vi "GOMBDTS2048 big sample.vi"() -> ()   [LabVIEW 2009]
uses:
  <vilib>/Utility/miscctls.llb/LVComboBoxStrsAndValuesArrayTypeDef.ctl
  <vilib>/Utility/file.llb/Write To Spreadsheet File (string).vi
panel:
  out "date/time string":string
  in  "Tab Control":T1(tab)
  in  "Configuration":string(combo)
  in  "Save Measurement":bool
  in  "Start Measurement":bool
  in  "Stop Software":bool
  in  "Initialize":bool
  out "XY Graph":cluster{"lambdas":dbl[], "counts":dbl[]}(graph)
  in  "X-Achse":enum16{"Wellenlänge / nm", "Pixel"}(ring)
  out "Filterposition":i32
  out "spectral unit":string
  out "integral unit":string
  out "x":dbl
  out "y":dbl
  out "T":dbl
  out "us":dbl
  out "vs":dbl
  out "domWL":dbl
  out "lambda peak":dbl
  out "fwhm":dbl
  out "scaling factor diode":dbl
  out "T / °C":dbl
  out "UpperX":dbl
  out "UpperY":dbl
  out "UpperZ":dbl
  out "Werte Y-Achse":dbl[](array[numeric])
  out "Werte X-Achse":dbl[](array[numeric])
  in  "Integrationszeit Automatisch?":bool=TRUE
  out "Integrationszeit / us":i32
  in  "Bandbreitenkorrektur":bool
  in  "Linearitätskorrektur":bool
  in  "a(Z)":bool
  in  "scale by diode":bool
  in  "Savitzky \nGolay Filter":bool
  out "az":dbl
  in  "Messmodus":T2(ring)
  in  "Anzahl Mittelungen":i32=1
  in  "Integrationszeit manuell / us":i32
  out "Temperature / °C":dbl
  in  "serial number device":string
  out "Integral value":dbl format="%#_6e"
  out "uv":dbl
  out "power peak":dbl
  out "handle":i32
  in  "Dateiname Selbstabsorptionskorrektur":string="sub1.gsc"
  in  "Selbstabsorptions-Korrektur nutzen?":bool
  in  "Speicherpfad Selbstabsorptions-Korrektur":path
  out "substititution factors array":dbl[](array[numeric])
  out "substitution factor diode":dbl
  out "function return 1":i32
  out "function return 3":i32
  out "Array function return 4":i32[](array[numeric])
  out "function return 5":i32
  out "function return 6":i32
  out "function return 7":i32
  out "function return 8":i32
  out "function return 14":i32
  out "function return 15":i32
  out "function return 16":i32
  out "function return 17":i32
  out "function return 19":i32
  out "function return 20":i32
  out "function return 21":i32
  out "function return 22":i32
  out "function return 23":i32
  out "function return 24":i32
  out "function return 25":i32
  out "function return 26":i32
  out "function return 27":i32
  out "function return 28":i32
  out "function return 29":i32
  out "function return 31":i32
  out "function return 34":i32
  out "function return 35":i32
  out "function return 36":i32
  out "function return 37":i32
  out "function return 38":i32
  out "function return 39":i32
  out "function return 40":i32
  out "function return 41":i32
  out "function return 43":i32
  out "function return 44":i32
  out "function return 45":i32
  out "function return 30":i32
  out "function return 33":i32
  out "function return 11":i32
  out "function return 10":i32
  out "function return 42":i32
  out "function return 32":i32
  out "function return 12":i32
  out "function return 13":i32
  out "function return 18":i32
  in  "error in":errorcluster
  out "error out":errorcluster
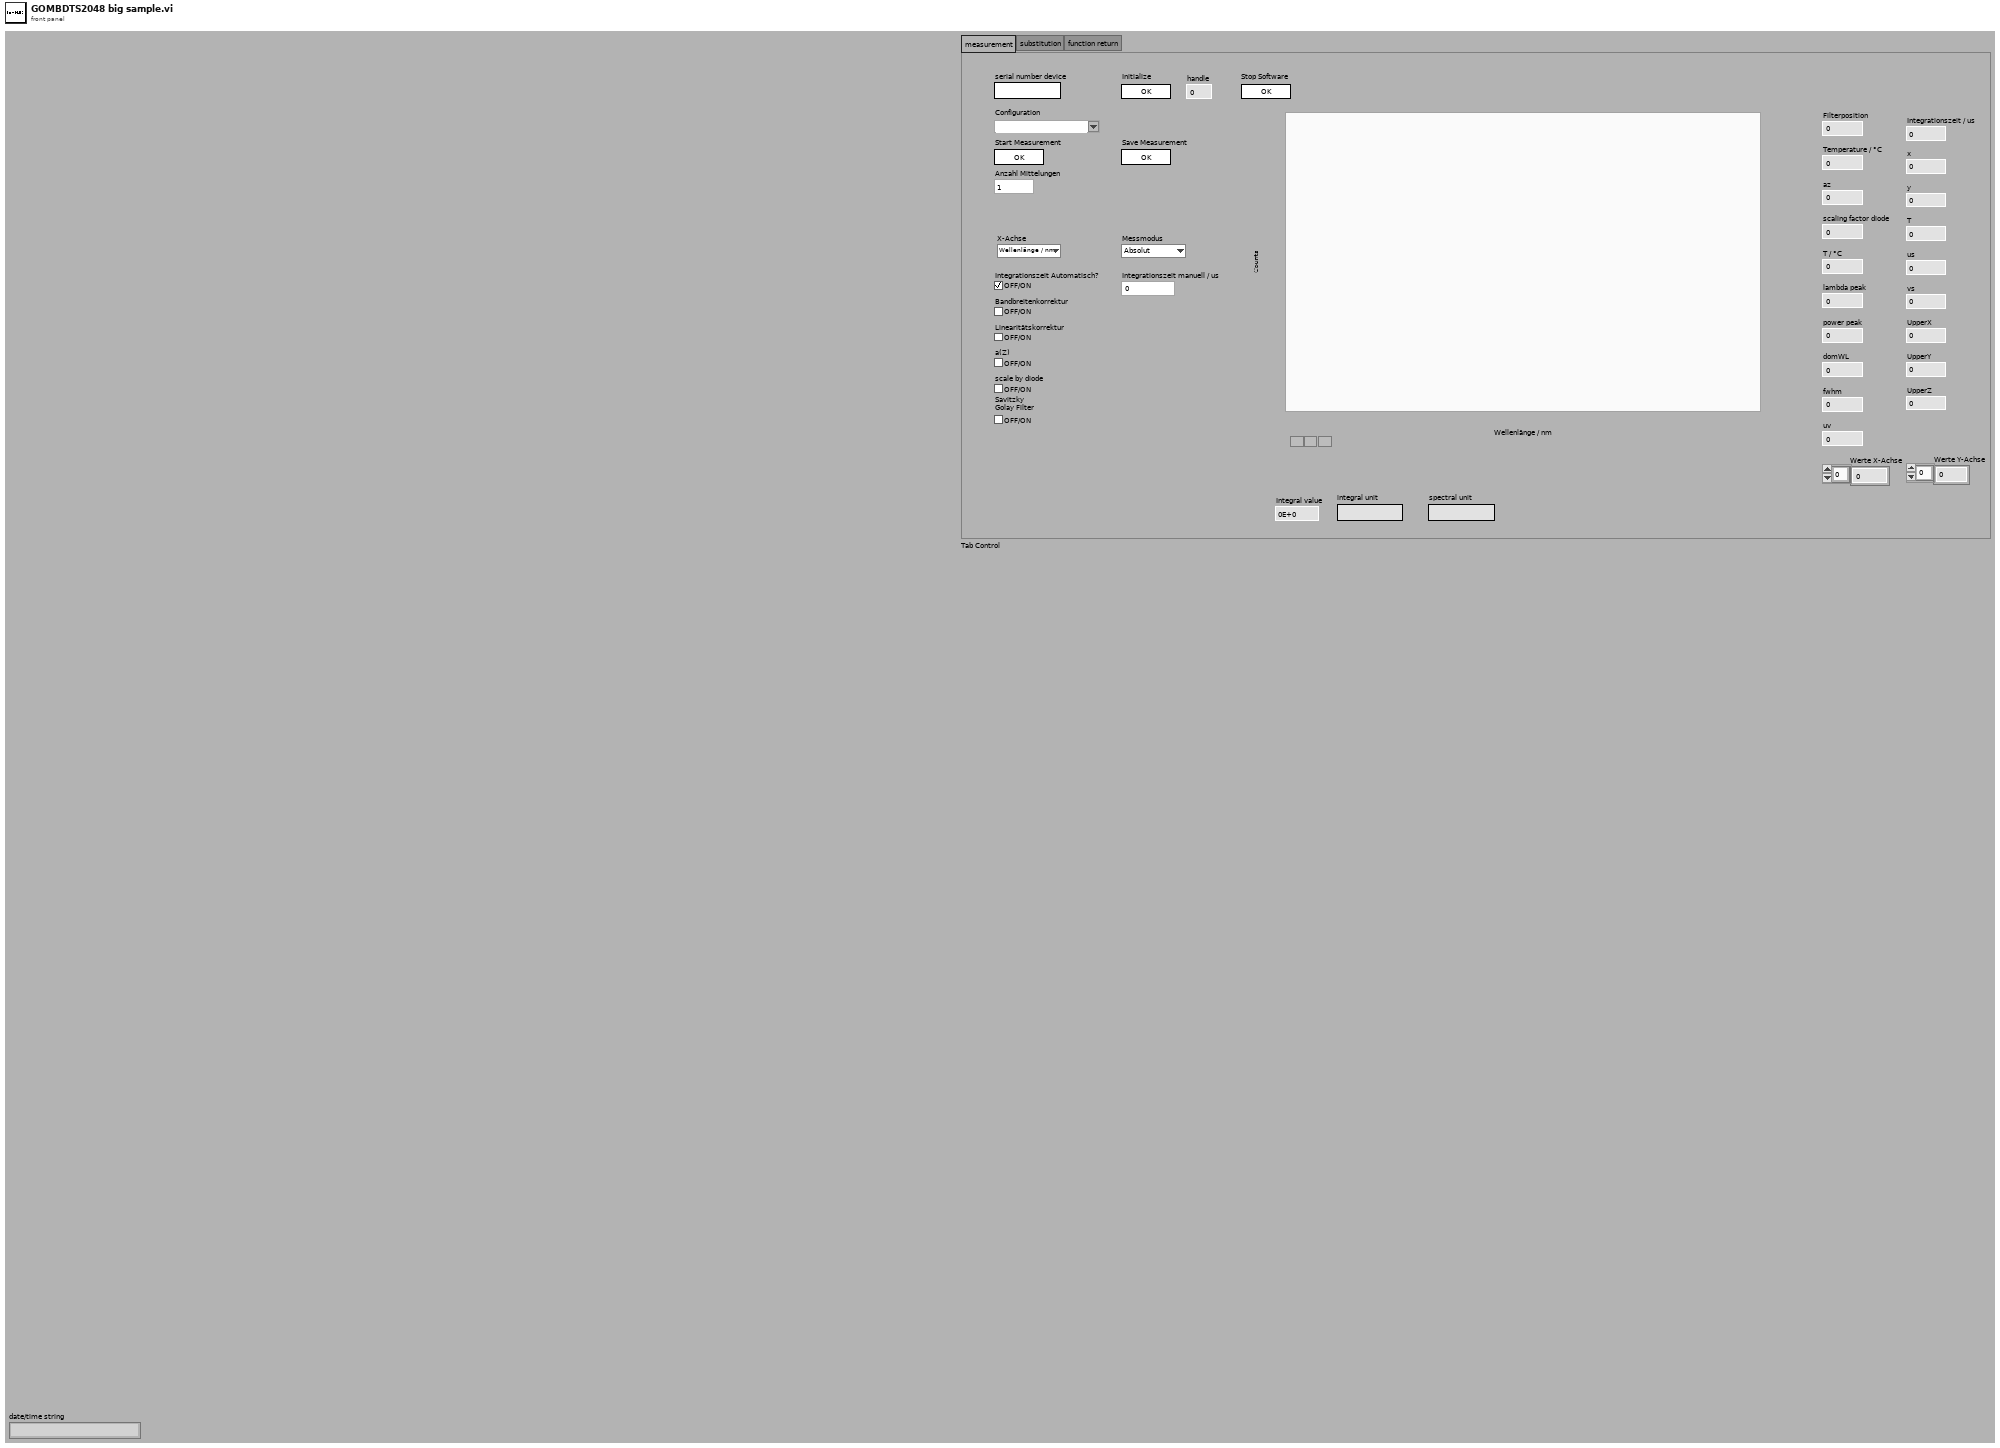
[diagram p1: front panel]
types:
  T1 = enum32{"measurement", "substitution", "function return"}
  T2 = enum16{"Absolut", "Counts", "Counts nur Hell", "Counts nur Dunkel"}
  T3 = typedef "LVComboBoxStrsAndValuesArrayTypeDef.ctl" = cluster{"String":string, "Value":string}[]
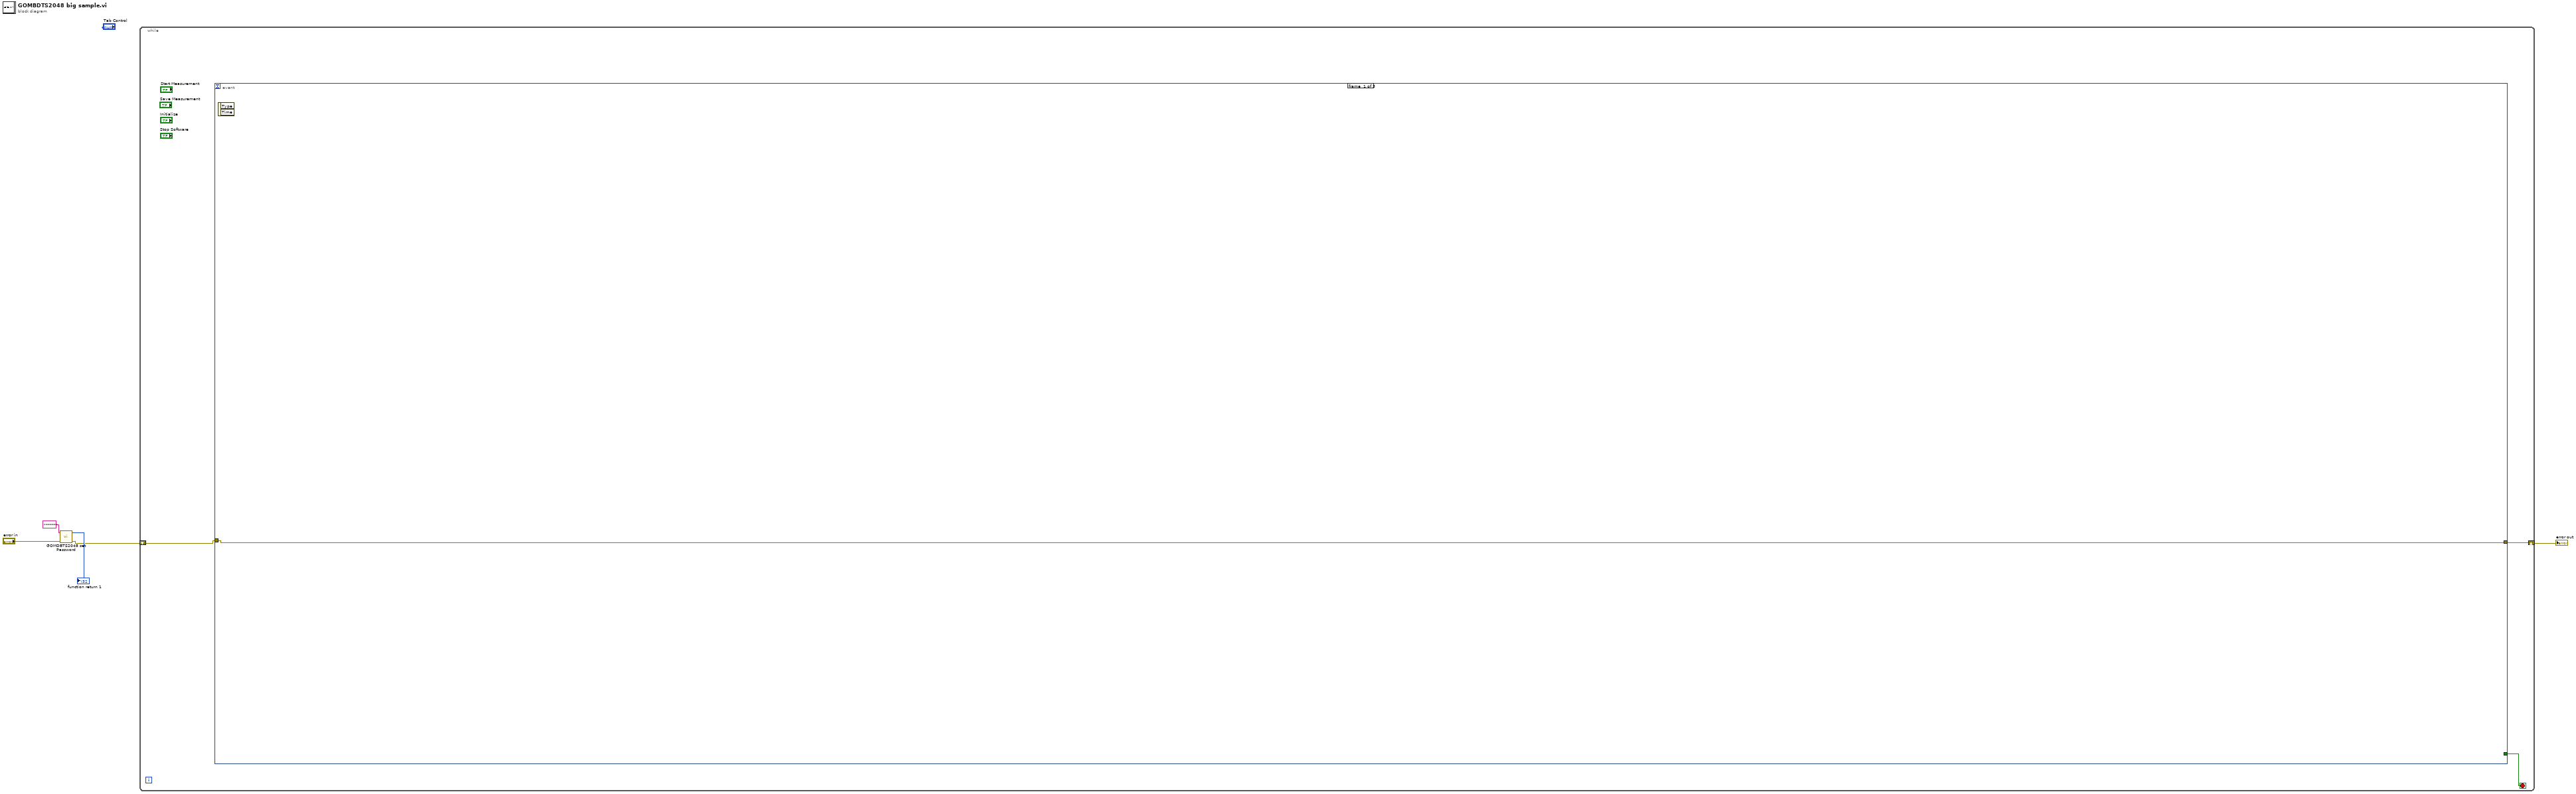
[diagram p0: block diagram]
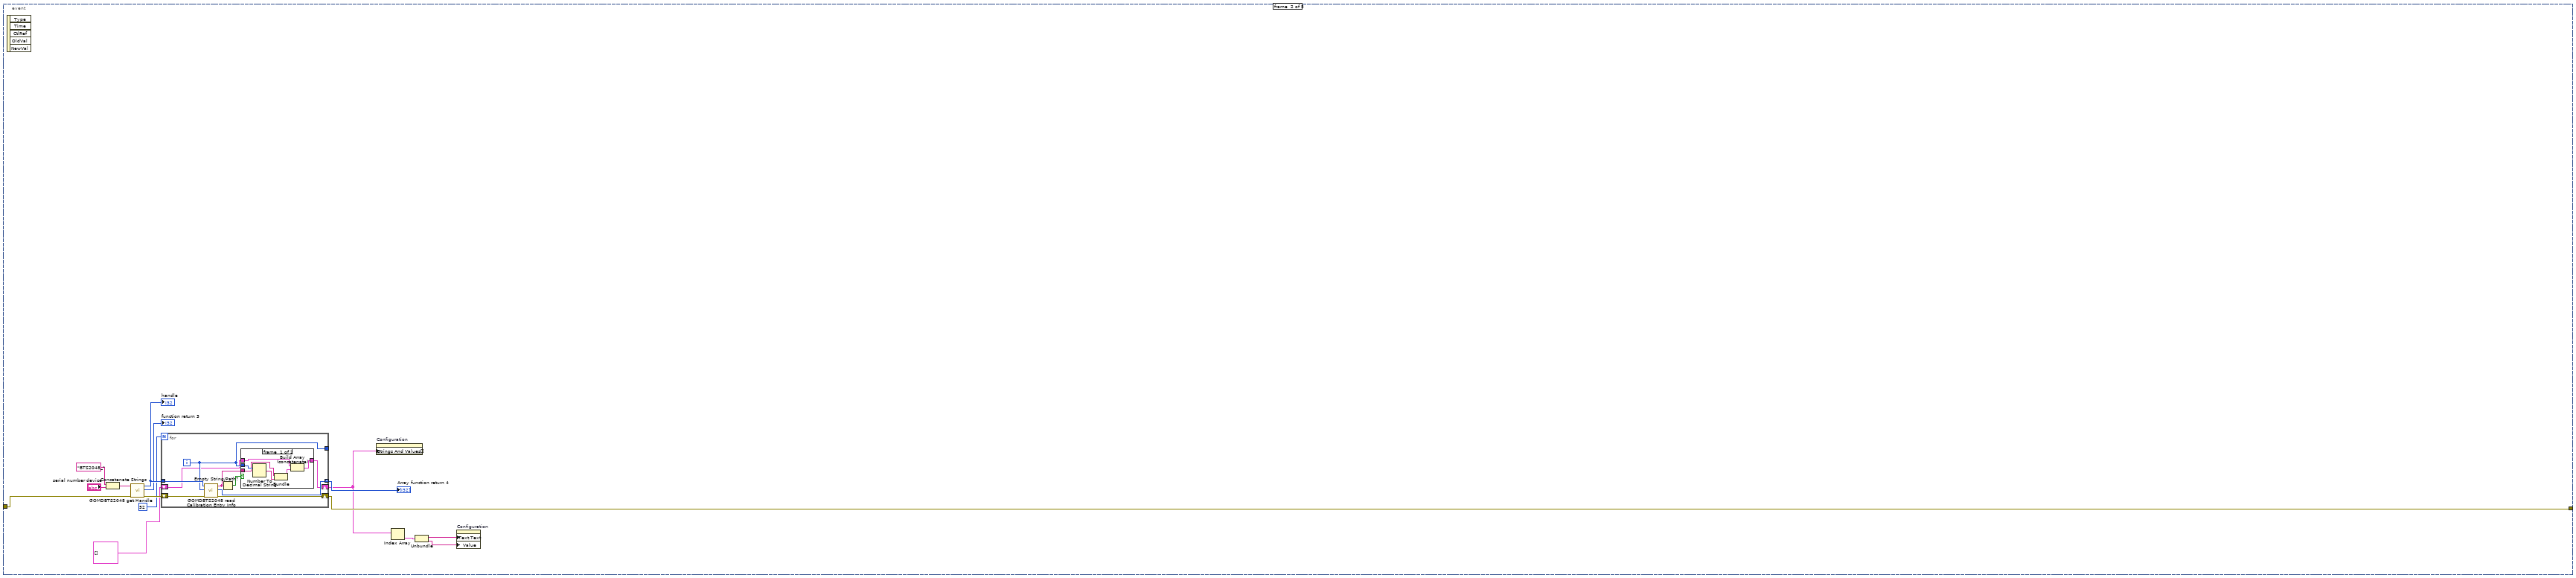
[diagram p2: hidden frame]
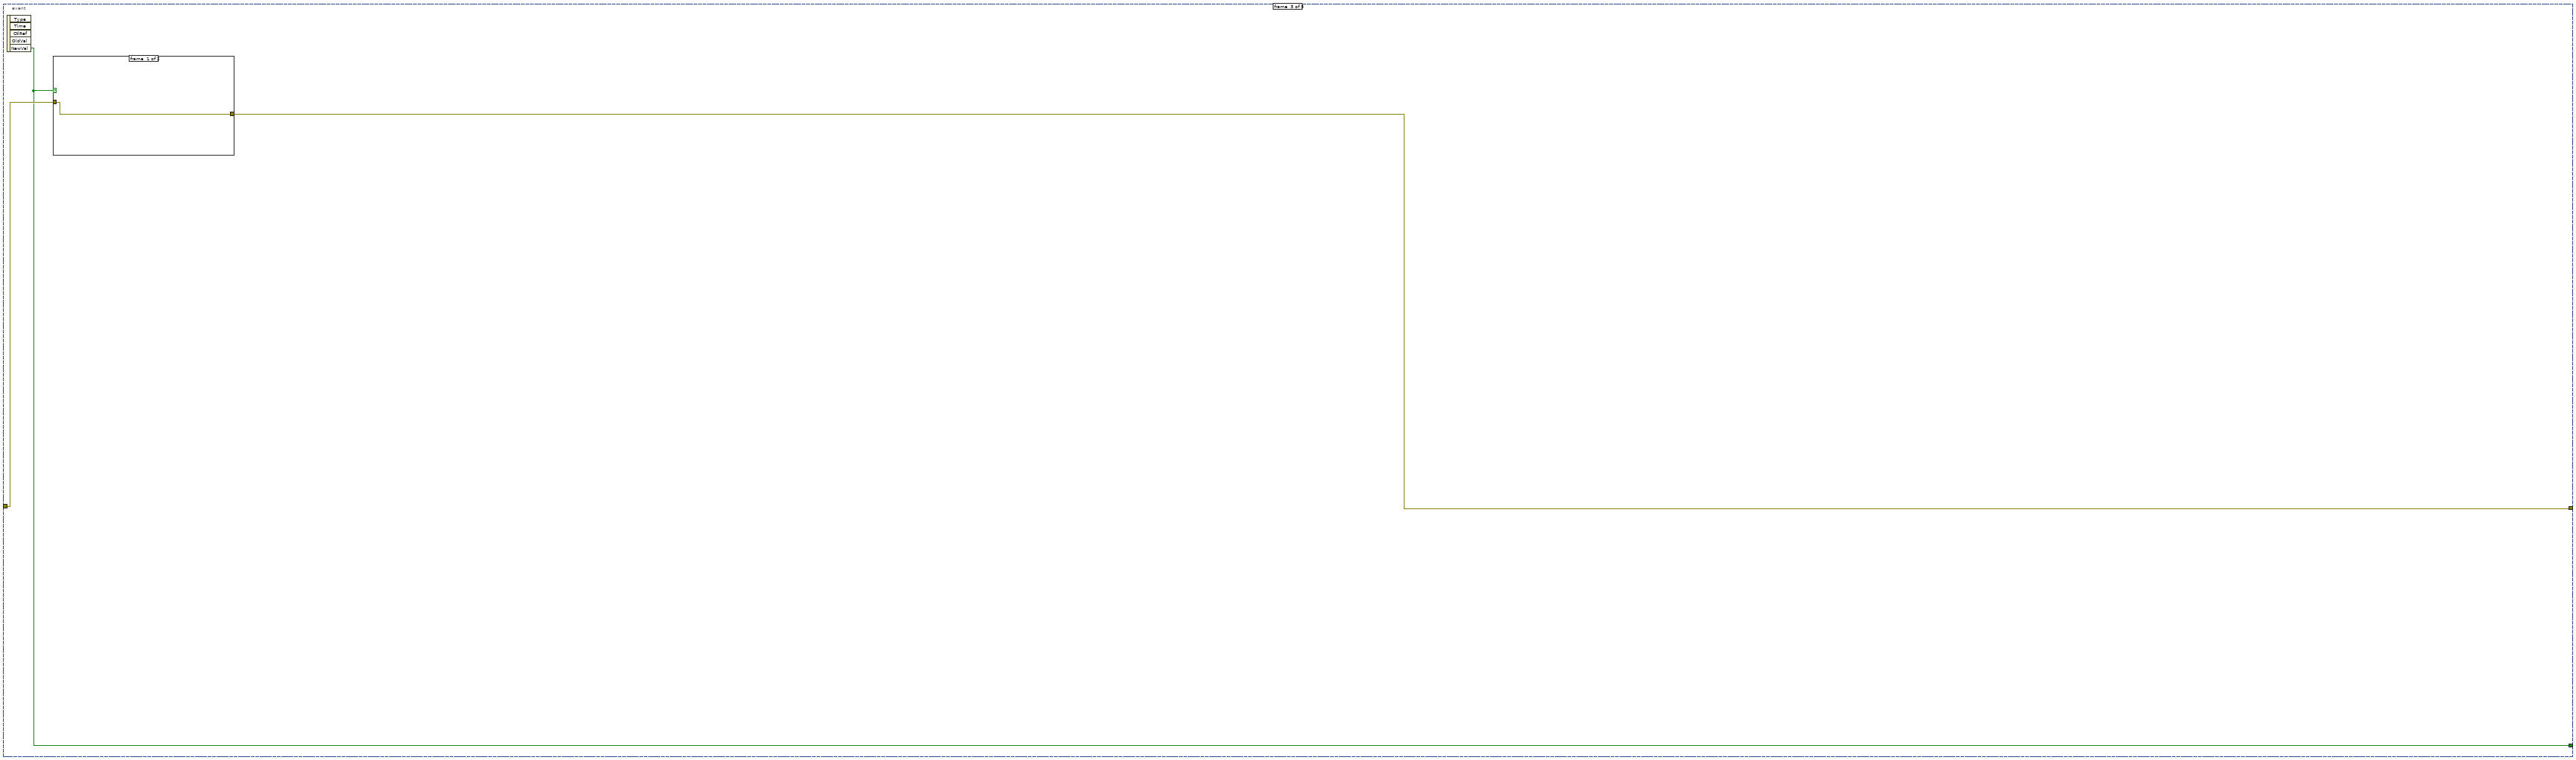
[diagram p4: hidden frame]
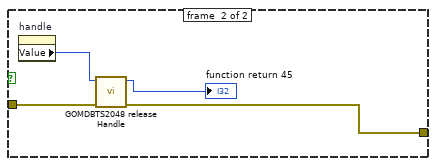
[diagram p5: hidden frame]
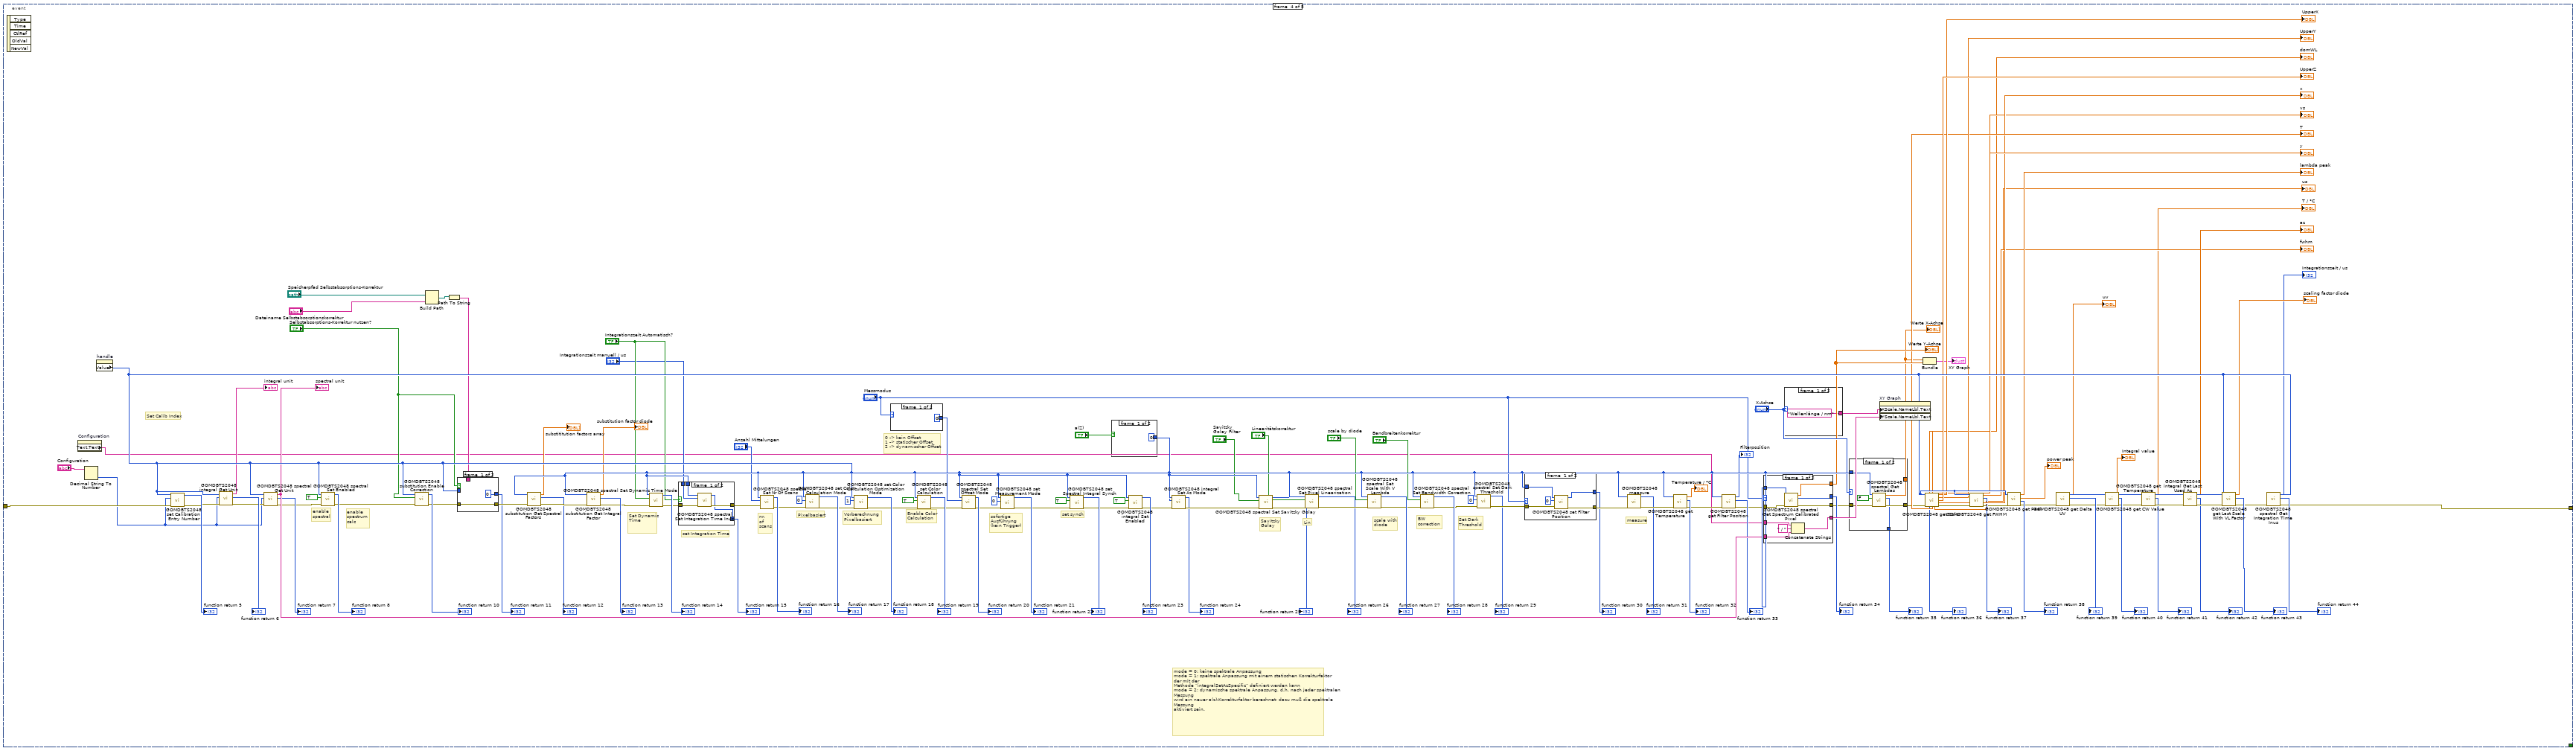
[diagram p6: hidden frame]
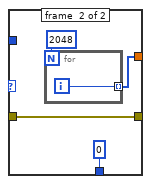
[diagram p7: hidden frame]
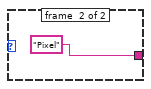
[diagram p8: hidden frame]
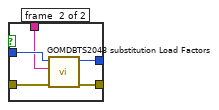
[diagram p9: hidden frame]
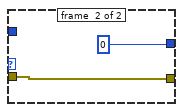
[diagram p10: hidden frame]
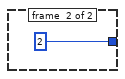
[diagram p11: hidden frame]
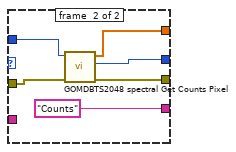
[diagram p12: hidden frame]
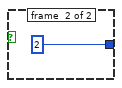
[diagram p13: hidden frame]
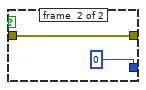
[diagram p14: hidden frame]
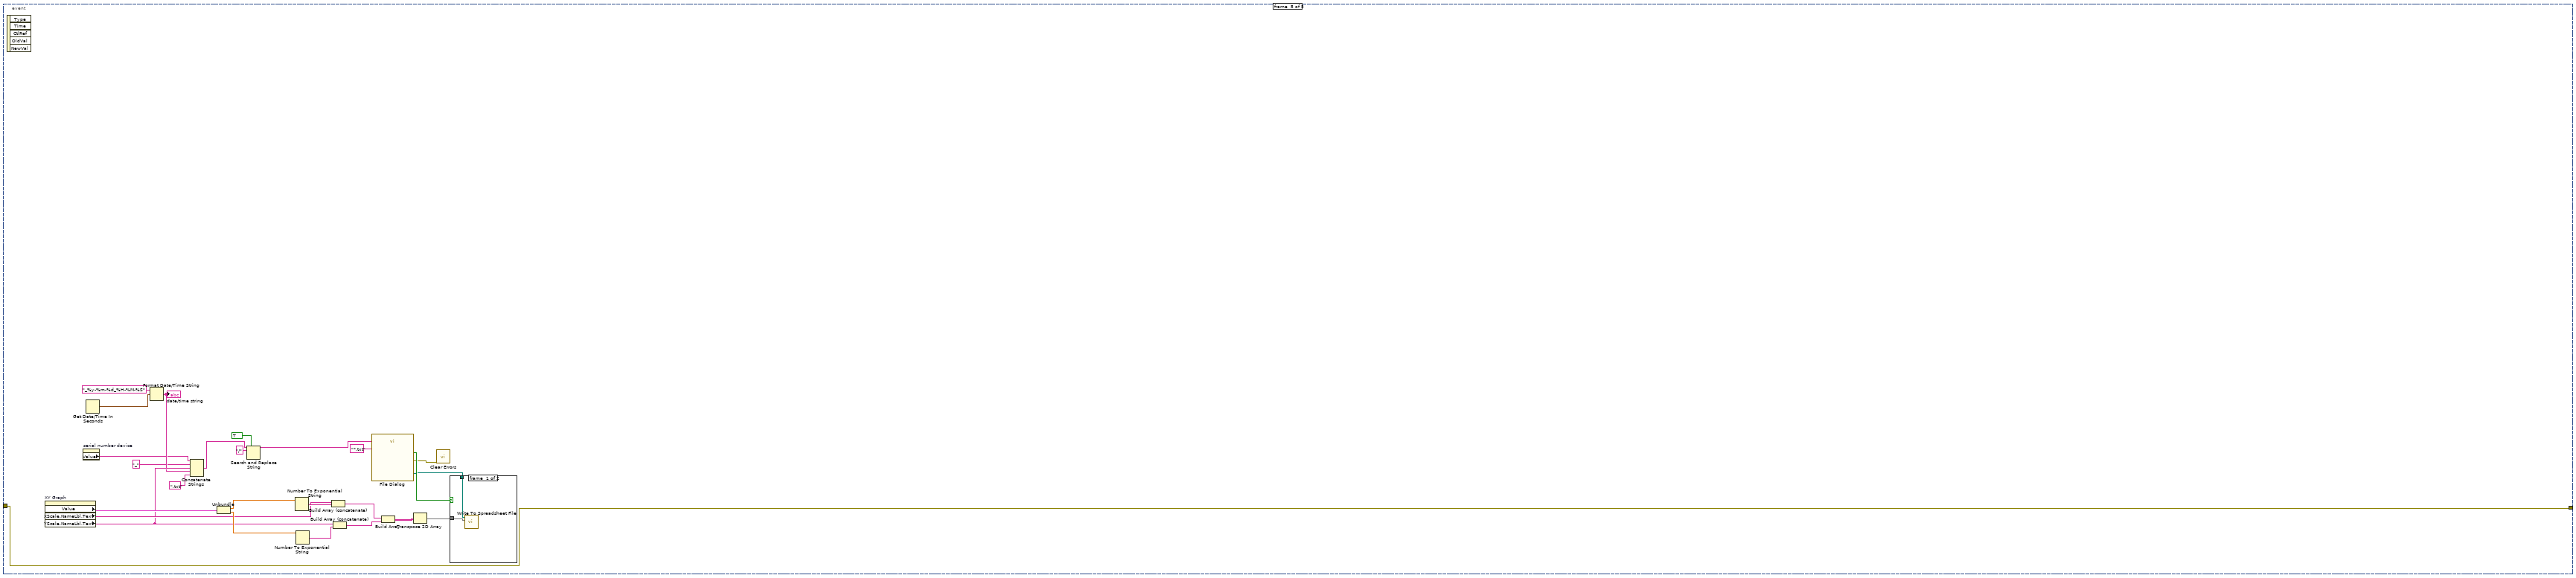
[diagram p15: hidden frame]
diagram:
  n1 = call <userlib>:"GOMDBTS2048 set Password.vi"("error in (no error)"="error in", "value"="*****" ("Password")) -> ("error out"=w2:errorcluster, "function return"=→"function return 1":i32)  [unwired: 8 in]
  n2 = while {
    shift-right: [w7] -> w1
    shift-left: w2 -> [w8]
    stop <- w6 stop-if-true
    n3 = event shown="[3] \"Start Measurement\": Value Change" {
      selector: _ -> [_ _ _ _ _]
      dyn-events: _ -> [_ _ _ _ _]
      timeout: _ -> [_ _ _ _ _]
      tunnel: w8 -> [w9 w16 w43 w57 w246]
      tunnel: [w9 w15 w42 w56 w246] -> w7
      tunnel: [_ _ w41 _ _] -> w6
      event #0 {
        n4 = event-data() -> ()  [unwired: 1 in, 2 out]
      }
      event #1 {
        n5 = event-data() -> ()  [unwired: 1 in, 5 out]
        n6 = Concatenate Strings("BTS2048_", "serial number device") -> (w18:string)
        n7 = call <userlib>:"GOMDBTS2048 get Handle.vi"("error in (no error)"=w16, "device"=w18) -> ("error out"=w20:errorcluster, "function return"=→"function return 3":i32, "handle"=w24:i32)  [unwired: 7 in]
        "handle" <- w24
        n8 = for {
          N: 52 -> [_]
          shift-right: [w31] -> w15
          shift-left: w20 -> [w32]
          tunnel: w24 -> [w33]
          tunnel: [w29] -> _
          tunnel: [w30] -> w22 mode=indexing
          shift-right: [w26] -> w13
          shift-left: T3 [] ("Strings And Values []") -> [w25]
          i -> [w29]
          n9 = call <userlib>:"GOMDBTS2048 read Calibration Entry Info.vi"("error in (no error)"=w32, "calibrationEntryNumber"=w29, "handle"=w33) -> ("error out"=w31:errorcluster, "function return"=w30:i32, "calibrationName"=w28:string)  [unwired: 6 in]
          n10 = Empty String/Path?(string/path=w28) -> (empty?=w27:bool)
          n11 = case shown="False" w27 {
            tunnel: w29 -> [w39 _]
            tunnel: w28 -> [w36 _]
            tunnel: [w37 w40] -> w26
            tunnel: w25 -> [w38 w40]
            frame #0 {
              n12 = Number To Decimal String(number=w39) -> (decimal integer string=w35:string)  [unwired: 1 in]
              n13 = Bundle("calibrationName"=w36, w35) -> (w34:cluster{"calibrationName":string, string})  [unwired: 1 in]
              n14 = Build Array (concatenate)(w38, w34) -> (w37:T3)
            }
            frame #1 {
            }
          }
        }
        "Array function return 4" <- w22
        n15 = property on="Configuration" class="CmbBox"("Strings And Values[]"=w13) -> ()  [unwired: 2 in, 2 out]
        n16 = Index Array(array=w13) -> (element=w12:cluster{"String":string, "Value":string})  [unwired: 1 in]
        n17 = Unbundle(w12) -> ("String"=w11:string, "Value"=w10:string)
        n18 = property on="Configuration" class="CmbBox"("Text.Text"=w11, "Value"=w10) -> ()  [unwired: 2 in, 2 out]
      }
      event #2 {
        n19 = event-data() -> ("NewVal"=w41:bool)  [unwired: 1 in, 4 out]
        n20 = case shown="True" w41 {
          tunnel: w43 -> [w44 w48]
          tunnel: [w44 w47] -> w42
          frame #0 {
          }
          frame #1 {
            n21 = property on="handle" class="DigNum (strict)"() -> ("Value"=w45:i32)  [unwired: 2 in, 2 out]
            n22 = call <userlib>:"GOMDBTS2048 release Handle.vi"("error in (no error)"=w48, "handle"=w45) -> ("error out"=w47:errorcluster, "function return"=→"function return 45":i32)  [unwired: 8 in]
          }
        }
      }
      event #3 {
        # "measure"
        # "Set Dark\nThreshold"
        # "BW \ncorrection"
        # "scale with\ndiode"
        # "Lin"
        # "Savitzky \nGolay"
        # "nr. \nof \nscans"
        # "enable\nspectrum\ncalc"
        # "enable\nspectral"
        # "set synch"
        # "sofortige\nAusführung\n(kein Trigger)"
        # "mode = 0: keine spektrale Anpassung\nmode = 1: spektrale Anpassung mit einem statischen Korrekturfaktor der mit der\nMethode “integralSetAzSpecific” definiert werden kann\nmode = 2: dynamische spektrale Anpassung, d.h. nach jeder spektralen Messung\nwird ein neuer a(z)-Korrekturfaktor berechnet; dazu muß die spektrale Messung\naktiviert sein."
        # "0 -> kein Offset\n1 -> statischer Offset\n2 -> dynamischer Offset"
        # "Set Calib Index"
        # "Set Dynamic Time"
        # "set Integration Time"
        # "Enable Color\nCalculation"
        # "Vorberechnung \nPixelbasiert"
        # "Pixelbasiert"
        n23 = event-data() -> ()  [unwired: 1 in, 5 out]
        n24 = property on="Configuration" class="CmbBox"() -> ("Text.Text"=w53:string)  [unwired: 2 in, 2 out]
        n25 = Decimal String To Number(string="Configuration") -> (number=w54:i32)  [unwired: 2 in, 1 out]
        n26 = property on="handle" class="DigNum (strict)"() -> ("Value"=w185:i32)  [unwired: 2 in, 2 out]
        n27 = call <userlib>:"GOMDBTS2048 set Calibration Entry Number.vi"("error in (no error)"=w57, "calibrationEntryNumber"=w54, "handle"=w185) -> ("error out"=w86:errorcluster, "function return"=→"function return 5":i32)  [unwired: 7 in]
        n28 = call <userlib>:"GOMDBTS2048 integral Get Unit.vi"("error in (no error)"=w86, "calibrationEntryNumber"=w54, "handle"=w185) -> ("error out"=w87:errorcluster, "function return"=→"function return 6":i32, "unit"=→"integral unit":string)  [unwired: 6 in]
        n29 = call <userlib>:"GOMDBTS2048 spectral Get Unit.vi"("error in (no error)"=w87, "calibrationEntryNumber"=w54, "handle"=w185) -> ("error out"=w88:errorcluster, "function return"=→"function return 7":i32, "unit"=w183:string)  [unwired: 6 in]
        "spectral unit" <- w183
        n30 = call <userlib>:"GOMDBTS2048 spectral Set Enabled.vi"("error in (no error)"=w88, "enabled"=TRUE, "handle"=w185) -> ("error out"=w49:errorcluster, "function return"=→"function return 8":i32)  [unwired: 7 in]
        n31 = call <userlib>:"GOMDBTS2048 substitution Enable Correction.vi"("error in (no error)"=w49, "active"="Selbstabsorptions-Korrektur nutzen?", "handle"=w185) -> ("error out"=w140:errorcluster, "function return"=→"function return 10":i32)  [unwired: 7 in]
        n32 = Build Path(base path="Speicherpfad Selbstabsorptions-Korrektur", name or relative path="Dateiname Selbstabsorptionskorrektur") -> (appended path=w143:path)
        n33 = Path To String(path=w143) -> (string=w144:string)
        n34 = case shown="True" "Selbstabsorptions-Korrektur nutzen?" {
          tunnel: w140 -> [w200 w205]
          tunnel: w185 -> [_ w204]
          tunnel: [w200 w203] -> w156
          tunnel: w144 -> [_ w202]
          tunnel: [0 ("function return") w201] -> w146
          frame #0 {
          }
          frame #1 {
            n35 = call <userlib>:"GOMDBTS2048 substitution Load Factors.vi"("error in (no error)"=w205, "absoluteFileName"=w202, "handle"=w204) -> ("error out"=w203:errorcluster, "function return"=w201:i32)  [unwired: 7 in]
          }
        }
        "function return 11" <- w146
        n36 = call <userlib>:"GOMDBTS2048 substitution Get Spectral Factors.vi"("error in (no error)"=w156, "handle"=w185) -> ("error out"=w159:errorcluster, "function return"=→"function return 12":i32, "factor"=→"substititution factors array":dbl[])  [unwired: 7 in]
        n37 = call <userlib>:"GOMDBTS2048 substitution Get Integral Factor.vi"("error in (no error)"=w159, "handle"=w185) -> ("error out"=w160:errorcluster, "function return"=→"function return 13":i32, "factor"=→"substitution factor diode":dbl)  [unwired: 7 in]
        n38 = call <userlib>:"GOMDBTS2048 spectral Set Dynamic Time Mode.vi"("error in (no error)"=w160, "value"="Integrationszeit Automatisch?", "handle"=w185) -> ("error out"=w64:errorcluster, "function return"=→"function return 14":i32)  [unwired: 7 in]
        n39 = case shown="True" "Integrationszeit Automatisch?" {
          tunnel: w64 -> [w236 w238]
          tunnel: [w235 w238] -> w80
          tunnel: w185 -> [w234 _]
          tunnel: "Integrationszeit manuell / us" -> [w233 _]
          tunnel: [w232 0 ("function return")] -> w107
          frame #0 {
            n40 = call <userlib>:"GOMDBTS2048 spectral Set Integration Time Inus.vi"("error in (no error)"=w236, "timeInus"=w233, "handle"=w234) -> ("error out"=w235:errorcluster, "function return"=w232:i32)  [unwired: 7 in]
          }
          frame #1 {
          }
        }
        "function return 15" <- w107
        n41 = call <userlib>:"GOMDBTS2048 spectral Set Nr Of Scans.vi"("error in (no error)"=w80, "value"="Anzahl Mittelungen", "handle"=w185) -> ("error out"=w81:errorcluster, "function return"=→"function return 16":i32)  [unwired: 7 in]
        n42 = call <userlib>:"GOMDBTS2048 set Color Calculation Mode.vi"("error in (no error)"=w81, "value"=0, "handle"=w185) -> ("error out"=w65:errorcluster, "function return"=→"function return 17":i32)  [unwired: 7 in]
        n43 = call <userlib>:"GOMDBTS2048 set Color Calculation Optimization Mode.vi"("error in (no error)"=w65, "value"=1, "handle"=w185) -> ("error out"=w66:errorcluster, "function return"=→"function return 18":i32)  [unwired: 7 in]
        n44 = case shown="\"Absolut\", \"Counts\"" "Messmodus" {
          tunnel: [0 ("mode") 2 ("mode")] -> w101
          frame #0 {
          }
          frame #1 {
          }
        }
        n45 = call <userlib>:"GOMDBTS2048 set Color Calculation.vi"("error in (no error)"=w66, "value"=TRUE, "handle"=w185) -> ("error out"=w70:errorcluster, "function return"=→"function return 19":i32)  [unwired: 7 in]
        n46 = call <userlib>:"GOMDBTS2048 spectral Set Offset Mode.vi"("error in (no error)"=w70, "value"=w101, "handle"=w185) -> ("error out"=w75:errorcluster, "function return"=→"function return 20":i32)  [unwired: 7 in]
        n47 = call <userlib>:"GOMDBTS2048 set Measurement Mode.vi"("error in (no error)"=w75, "measurementMode"=0, "handle"=w185) -> ("error out"=w77:errorcluster, "function return"=→"function return 21":i32)  [unwired: 7 in]
        n48 = call <userlib>:"GOMDBTS2048 set Spectral Integral Synch.vi"("error in (no error)"=w77, "value"=TRUE, "handle"=w185) -> ("error out"=w78:errorcluster, "function return"=→"function return 22":i32)  [unwired: 7 in]
        n49 = case shown="True" "a(Z)" {
          tunnel: [0 ("mode") 2 ("mode")] -> w74
          frame #0 {
          }
          frame #1 {
          }
        }
        n50 = call <userlib>:"GOMDBTS2048 integral Set Enabled.vi"("error in (no error)"=w78, "enabled"=TRUE, "handle"=w185) -> ("error out"=w73:errorcluster, "function return"=→"function return 23":i32)  [unwired: 7 in]
        n51 = call <userlib>:"GOMDBTS2048 integral Set Az Mode.vi"("error in (no error)"=w73, "mode"=w74, "handle"=w185) -> ("error out"=w175:errorcluster, "function return"=→"function return 24":i32)  [unwired: 7 in]
        n52 = call <userlib>:"GOMDBTS2048 spectral Set Savitzky Golay.vi"("error in (no error)"=w175, "value"="Savitzky \nGolay Filter", "handle"=w185) -> ("error out"=w82:errorcluster, "function return"=→"function return 25":i32)  [unwired: 7 in]
        n53 = call <userlib>:"GOMDBTS2048 spectral Set Pixel Linearization.vi"("error in (no error)"=w82, "value"="Linearitätskorrektur", "handle"=w185) -> ("error out"=w163:errorcluster, "function return"=→"function return 26":i32)  [unwired: 7 in]
        n54 = call <userlib>:"GOMDBTS2048 spectral Set Scale With V Lambda.vi"("error in (no error)"=w163, "value"="scale by diode", "handle"=w185) -> ("error out"=w83:errorcluster, "function return"=→"function return 27":i32)  [unwired: 7 in]
        n55 = call <userlib>:"GOMDBTS2048 spectral Set Bandwidth Correction.vi"("error in (no error)"=w83, "value"="Bandbreitenkorrektur", "handle"=w185) -> ("error out"=w84:errorcluster, "function return"=→"function return 28":i32)  [unwired: 7 in]
        n56 = call <userlib>:"GOMDBTS2048 spectral Set Dark Threshold.vi"("error in (no error)"=w84, "value"=0, "handle"=w185) -> ("error out"=w134:errorcluster, "function return"=→"function return 29":i32)  [unwired: 7 in]
        n57 = case shown="\"Counts nur Dunkel\"" "Messmodus" {
          tunnel: w134 -> [w210 w212]
          tunnel: [w209 w212] -> w151
          tunnel: w185 -> [w208 _]
          tunnel: [w206 0 ("function return")] -> w135
          frame #0 {
            n58 = call <userlib>:"GOMDBTS2048 set Filter Position.vi"("error in (no error)"=w210, "value"=0, "handle"=w208) -> ("error out"=w209:errorcluster, "function return"=w206:i32)  [unwired: 7 in]
          }
          frame #1 {
          }
        }
        "function return 30" <- w135
        n59 = call <userlib>:"GOMDBTS2048 measure.vi"("error in (no error)"=w151, "handle"=w185) -> ("error out"=w152:errorcluster, "function return"=→"function return 31":i32)  [unwired: 8 in]
        n60 = call <userlib>:"GOMDBTS2048 get Temperature.vi"("error in (no error)"=w152, "handle"=w185) -> ("error out"=w153:errorcluster, "function return"=→"function return 32":i32, "value"=→"Temperature / °C":dbl)  [unwired: 7 in]
        n61 = call <userlib>:"GOMDBTS2048 get Filter Position.vi"("error in (no error)"=w153, "handle"=w185) -> ("error out"=w136:errorcluster, "function return"=→"function return 33":i32, "value"=→"Filterposition":i32)  [unwired: 7 in]
        n62 = case shown="\"Counts\"..\"Counts nur Dunkel\"" "Messmodus" {
          tunnel: w136 -> [w223 w229]
          tunnel: [w222 w228] -> w89
          tunnel: w185 -> [w221 w227]
          tunnel: [w220 w226] -> w181
          tunnel: [w219 w225] -> w122
          tunnel: [w215 "Counts"] -> w180
          tunnel: w53 -> [w218 _]
          tunnel: w183 -> [w216 _]
          frame #0 {
            n63 = call <userlib>:"GOMDBTS2048 spectral Get Spectrum Calibrated Pixel.vi"("error in (no error)"=w223, "handle"=w221) -> ("error out"=w222:errorcluster, "function return"=w219:i32, "spectrum"=w220:dbl[])  [unwired: 7 in]
            n64 = Concatenate Strings(w218, " / " ("string"), w216) -> (w215:string)
          }
          frame #1 {
            n65 = call <userlib>:"GOMDBTS2048 spectral Get Counts Pixel.vi"("error in (no error)"=w229, "handle"=w227) -> ("error out"=w228:errorcluster, "function return"=w225:i32, "counts"=w226:dbl[])  [unwired: 7 in]
          }
        }
        "Werte Y-Achse" <- w181
        "function return 34" <- w122
        n66 = case shown="\"Wellenlänge / nm\", Default" "X-Achse" {
          tunnel: ["Wellenlänge / nm" "Pixel"] -> w184
          frame #0 {
          }
          frame #1 {
          }
        }
        n67 = case shown="\"Pixel\"" "X-Achse" {
          tunnel: w89 -> [w191 w194]
          tunnel: [w190 w194] -> w90
          tunnel: [w189 0 ("function return")] -> w123
          tunnel: [w187 w192] -> w131
          tunnel: w185 -> [w186 _]
          frame #0 {
            n68 = call <userlib>:"GOMDBTS2048 spectral Get Lambdas.vi"("error in (no error)"=w191, "wavelengthRaster"=FALSE, "handle"=w186) -> ("error out"=w190:errorcluster, "function return"=w189:i32, "lambdas"=w187:dbl[])  [unwired: 6 in]
          }
          frame #1 {
            n69 = for {
              N: 2048 -> [_]
              tunnel: [w196] -> w192 mode=indexing
              i -> [w196]
            }
          }
        }
        "Werte X-Achse" <- w131
        "function return 35" <- w123
        n70 = property on="XY Graph" class="XYGraph (strict)"("XScale.NameLbl.Text"=w184, "YScale.NameLbl.Text"=w180) -> ()  [unwired: 2 in, 2 out]
        n71 = Bundle("lambdas"=w131, "counts"=w181) -> (→"XY Graph":cluster{"lambdas":dbl[], "counts":dbl[]})  [unwired: 1 in]
        n72 = call <userlib>:"GOMDBTS2048 get Color.vi"("handle"=w185, "error in (no error)"=w90) -> ("domWL"=→"domWL":dbl, "vs"=→"vs":dbl, "y"=→"y":dbl, "UpperX"=→"UpperX":dbl, "UpperY"=→"UpperY":dbl, "UpperZ"=→"UpperZ":dbl, "x"=→"x":dbl, "function return"=→"function return 36":i32, "CCT"=→"T":dbl, "us"=→"us":dbl, "error out"=w93:errorcluster)  [unwired: 3 in]
        n73 = call <userlib>:"GOMDBTS2048 get FWHM.vi"("error in (no error)"=w93, "handle"=w185) -> ("error out"=w95:errorcluster, "function return"=→"function return 37":i32, "fwhm"=→"fwhm":dbl)  [unwired: 7 in]
        n74 = call <userlib>:"GOMDBTS2048 get Peak.vi"("error in (no error)"=w95, "handle"=w185) -> ("error out"=w97:errorcluster, "function return"=→"function return 38":i32, "power"=→"power peak":dbl, "lambda"=→"lambda peak":dbl)  [unwired: 6 in]
        n75 = call <userlib>:"GOMDBTS2048 get Delta UV.vi"("error in (no error)"=w97, "handle"=w185) -> ("error out"=w98:errorcluster, "function return"=→"function return 39":i32, "uv"=→"uv":dbl)  [unwired: 7 in]
        n76 = call <userlib>:"GOMDBTS2048 get CW Value.vi"("error in (no error)"=w98, "handle"=w185) -> ("error out"=w99:errorcluster, "function return"=→"function return 40":i32, "value"=→"Integral value":dbl)  [unwired: 7 in]
        n77 = call <userlib>:"GOMDBTS2048 get Temperature.vi"("error in (no error)"=w99, "handle"=w185) -> ("error out"=w147:errorcluster, "function return"=→"function return 41":i32, "value"=→"T / °C":dbl)  [unwired: 7 in]
        n78 = call <userlib>:"GOMDBTS2048 integral Get Last Used Az.vi"("error in (no error)"=w147, "handle"=w185) -> ("error out"=w176:errorcluster, "function return"=→"function return 42":i32, "az"=→"az":dbl)  [unwired: 7 in]
        n79 = call <userlib>:"GOMDBTS2048 get Last Scale With VL Factor.vi"("error in (no error)"=w176) -> ("error out"=w177:errorcluster, "function return"=→"function return 43":i32, "value"=→"scaling factor diode":dbl)  [unwired: 8 in]
        n80 = call <userlib>:"GOMDBTS2048 spectral Get Integration Time Inus.vi"("error in (no error)"=w177, "handle"=w185) -> ("error out"=w56:errorcluster, "function return"=→"function return 44":i32, "timeInus"=→"Integrationszeit / us":i32)  [unwired: 7 in]
      }
      event #4 {
        n81 = event-data() -> ()  [unwired: 1 in, 5 out]
        n82 = property on="XY Graph" class="XYGraph (strict)"() -> ("Value"=w264:cluster{"lambdas":dbl[], "counts":dbl[]}, "XScale.NameLbl.Text"=w259:string, "YScale.NameLbl.Text"=w252:string)  [unwired: 2 in, 2 out]
        n83 = property on="serial number device" class="Str"() -> ("Value"=w248:string)  [unwired: 2 in, 2 out]
        n84 = Get Date/Time In Seconds() -> (seconds since 1Jan1904=w251:timestamp)
        n85 = Format Date/Time String(time format string (%c)="_%y-%m-%d_%H-%M-%S", seconds (now)=w251) -> (date/time string=w249:string)  [unwired: 1 in]
        "date/time string" <- w249
        n86 = Concatenate Strings(w248, "_" ("string"), w252, w249, ".txt" ("string")) -> (w242:string)
        n87 = Unbundle(w264) -> ("lambdas"=w263:dbl[], "counts"=w262:dbl[])
        n88 = Search and Replace String(replace all?=TRUE ("replace all? (F)"), input string=w242, search string="/") -> (result string=w239:string)  [unwired: 5 in, 3 out]
        n89 = Number To Exponential String(number=w263) -> (E-format string=w261:string[])  [unwired: 3 in]
        n90 = Number To Exponential String(number=w262) -> (E-format string=w260:string[])  [unwired: 3 in]
        n91 = Build Array (concatenate)(w259, w261) -> (w258:string[])
        n92 = Build Array (concatenate)(w252, w260) -> (w257:string[])
        n93 = call "File Dialog"("default name"=w239, "pattern (all files)"="*.txt") -> ("selected path"=w244:path, "cancelled"=w254:bool, "error out"=w245:errorcluster)  [unwired: 10 in, 1 out]
        n94 = Build Array(w258, w257) -> (w256:string[][])
        n95 = Transpose 2D Array(2D array=w256) -> (transposed array=w255:string[][])
        n96 = call <vilib>:"Clear Errors.vi"("error in (no error)"=w245) -> ()  [unwired: 6 in, 1 out]
        n97 = case shown="False" w254 {
          tunnel: w255 -> [w266 _]
          tunnel: w244 -> [w265 _]
          frame #0 {
            n98 = call-poly <vilib>:"Write To Spreadsheet File.vi"("2D data"=w266, "file path (dialog if empty)"=w265) -> ()  [unwired: 6 in, 1 out]
          }
          frame #1 {
          }
        }
      }
    }
  }
  "error out" <- w1
